vi "Weather Station UI.vi"(7 "정지":bool caption="stop", 9 "하위 리미트":dbl=10.0 min=0.0 max=50.0, 10 "상위 리미트":dbl=30.0 min=0.0 max=50.0) -> (1 "경고":string, 2 "온도 히스토리":dbl(graph))   [LabVIEW 2018]
doc: "이것은 기상 관측기 프로젝트의 주요 VI입니다. 이 VI에는 온도 경고 시스템을 위한 사용자 인터페이스가 있습니다. \n\n사용자 입력: 최고 온도, 최저 온도, 온도 단위\n출력: 현재 온도, 경고 상태"
uses:
  Supporting Files/Weather Station States.ctl
  Instance           1 26Saved   Weather Station UI .vi
panel:
  # "온도 범위"
  # "열사병"
  # "동상"
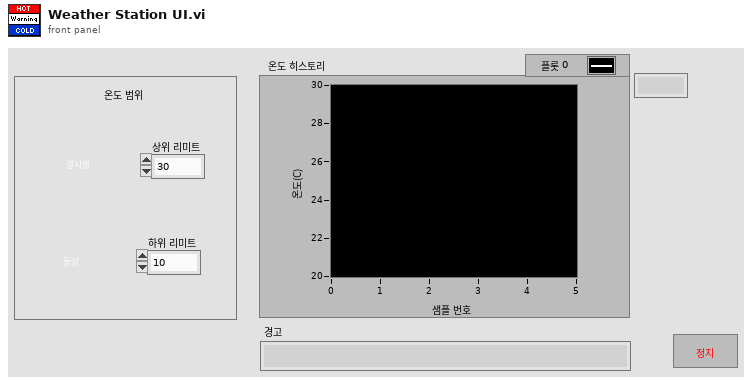
[diagram p1: front panel]
types:
  T1 = enum16{"open", "replace", "create", "open or create", "replace or create", "replace or create with confirmation"}
  T2 = typedef "Weather Station States.ctl" = enum16{"수집", "분석", "데이터 로그", "시간 확인"}
  T3 = cluster{"온도":dbl, "온도 상위 리미트":dbl, "온도 하위 리미트":dbl, "경고":string}
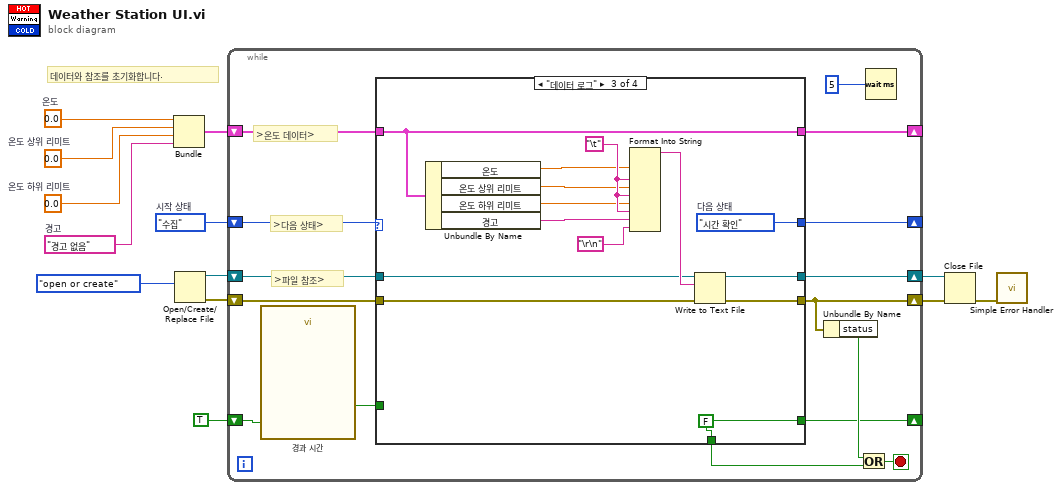
[diagram p0: block diagram]
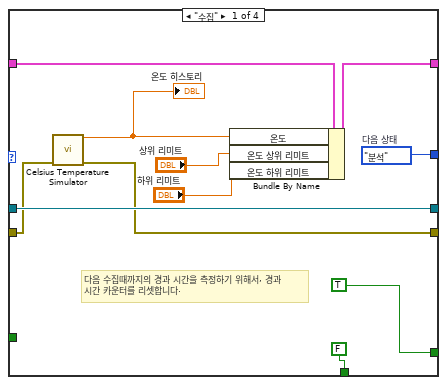
[diagram p2: hidden frame]
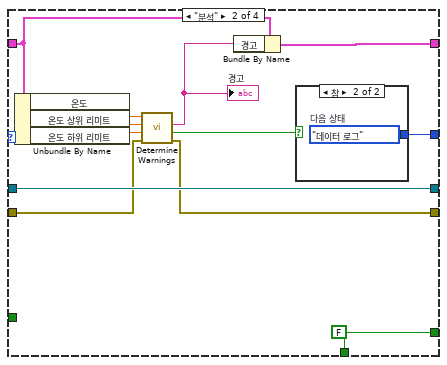
[diagram p3: hidden frame]
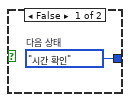
[diagram p4: hidden frame]
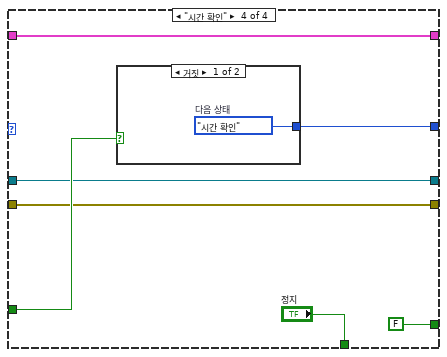
[diagram p5: hidden frame]
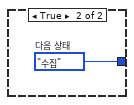
[diagram p6: hidden frame]
diagram:
  w7 = 0.0  # 온도 하위 리미트
  w6 = 0.0  # 온도 상위 리미트
  w8 = "경고 없음"  # 경고
  w4 = 0.0  # 온도
  w13 = Weather_Station_States."수집"  # 시작 상태
  # "데이터와 참조를 초기화합니다."
  n1 = Bundle("온도"=w4, "온도 상위 리미트"=w6, "온도 하위 리미트"=w7, "경고"=w8) -> (w1:T3)  [unwired: 1 in]
  n2 = Open/Create/Replace File(operation (0:open)=T1."open or create") -> (refnum out=w3:refnum<file>, error out=w2:errorcluster)  [unwired: 5 in, 1 out]
  n3 = while {
    shift-right: [w27] -> _
    shift-left: w13 -> [w28]
    shift-right: [w24] -> w12
    shift-left: w2 -> [w26]
    shift-right: [w14] -> _
    shift-left: w1 -> [w21]
    shift-right: [w22] -> w11
    shift-left: w3 -> [w20]
    shift-right: [w15] -> _
    shift-left: TRUE ("stop") -> [w17]
    stop <- w25 stop-if-true
    # ">온도 데이터>"
    # ">파일 참조>"
    # ">다음 상태>"
    n4 = call "경과 시간"("Reset"=w17) -> ("Time has Elapsed"=w16:bool)  [unwired: 11 in, 7 out]
    n5 = case shown="\"데이터 로그\"" w28 {
      tunnel: [w39 w49 w67 w73] -> w27
      tunnel: [w29 w42 w65 w69] -> w24
      tunnel: w26 -> [w30 w43 w66 w69]
      tunnel: [w38 w51 w64 w70] -> w22
      tunnel: [w32 w44 w54 w68] -> w14
      tunnel: w21 -> [w35 w45 w54 w68]
      tunnel: w20 -> [w38 w51 w62 w70]
      tunnel: [FALSE ("stop") w50 w60 "정지"] -> w19
      tunnel: w16 -> [_ _ _ w74]
      tunnel: [TRUE ("stop") w50 w60 FALSE ("stop")] -> w15
      frame "수집" {
        w39 = Weather_Station_States."분석"  # 다음 상태
        # "다음 수집때까지의 경과 시간을 측정하기 위해서, 경과 시간 카운터를 리셋합니다."
        n6 = call "Celsius Temperature Simulator.vi"("에러 입력(에러 없음)"=w30) -> ("온도"=w31:dbl, "에러 출력"=w29:errorcluster)  [unwired: 13 in]
        "온도 히스토리" <- w31
        n7 = Bundle By Name(cluster=w35, "온도"=w31, "온도 상위 리미트"="상위 리미트", "온도 하위 리미트"="하위 리미트") -> (w32:T3)
      }
      frame "분석" {
        w50 = FALSE ("stop")
        n8 = Unbundle By Name(w45) -> ("온도"=w48:dbl, "온도 상위 리미트"=w47:dbl, "온도 하위 리미트"=w46:dbl)
        n9 = call "Determine Warnings.vi"("에러 입력(에러 없음)"=w43, "최저 온도"=w46, "최고 온도"=w47, "현재 온도"=w48) -> ("에러 출력"=w42:errorcluster, "경고?"=w40:bool, "경고 텍스트"=w41:string)  [unwired: 5 in]
        "경고" <- w41
        n10 = Bundle By Name(cluster=w45, "경고"=w41) -> (w44:T3)
        n11 = case shown="참" w40 {
          tunnel: [w52 w53] -> w49
          frame False {
            w52 = Weather_Station_States."시간 확인"  # 다음 상태
          }
          frame True {
            w53 = Weather_Station_States."데이터 로그"  # 다음 상태
          }
        }
      }
      frame "데이터 로그" {
        w67 = Weather_Station_States."시간 확인"  # 다음 상태
        w60 = FALSE ("stop")
        w61 = "\t"
        n12 = Unbundle By Name(w54) -> ("온도"=w59:dbl, "온도 상위 리미트"=w58:dbl, "온도 하위 리미트"=w57:dbl, "경고"=w56:string)
        n13 = Format Into String(w59, w61, w58, w61, w57, w61, w56, "\r\n") -> (resulting string=w63:string)  [unwired: 3 in, 1 out]
        n14 = Write to Text File(file (use dialog)=w62, text=w63, error in=w66) -> (refnum out=w64:refnum<file>, error out=w65:errorcluster)  [unwired: 1 in, 1 out]
      }
      frame "시간 확인" {
        n15 = case shown="거짓" w74 {
          tunnel: [w75 w76] -> w73
          frame False {
            w75 = Weather_Station_States."시간 확인"  # 다음 상태
          }
          frame True {
            w76 = Weather_Station_States."수집"  # 다음 상태
          }
        }
      }
    }
    n16 = Unbundle By Name(w24) -> ("status"=w23:bool)
    n17 = Or(x=w23, y=w19) -> (x .or. y?=w25:bool)
    n18 = Wait (ms)(milliseconds to wait=u32 5 ("y")) -> ()  [unwired: 1 out]
  }
  n19 = Close File(refnum=w11, error in=w12) -> (error out=w10:errorcluster)  [unwired: 1 out]
  n20 = call <vilib>:"Simple Error Handler.vi"("error in (no error)"=w10) -> ()  [unwired: 4 in, 5 out]
